vi "CommandWrite.vi"(8 "error in (no error)":errorcluster, 10 "Write Buffer":string, 11 "VISA resource name":refnum<visa-resource-name>) -> (0 "error out":errorcluster, 3 "VISA resource name out":refnum<visa-resource-name>)   [LabVIEW 2020, in "LitePoints.lvlib"]
uses:
  LitePoints.lvlib
panel:
  out "output string":string
  out "Return Count":u32
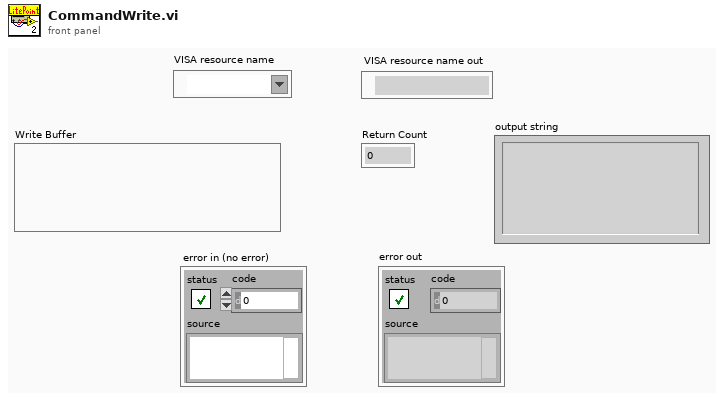
[diagram p1: front panel]
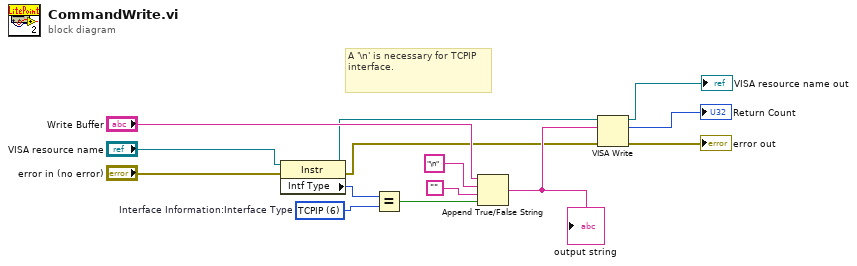
[diagram p0: block diagram]
diagram:
  w7 = u16 6 items=["GPIB"=1, "VXI"=2, "GPIB-VXI"=3, "Serial"=4, "PXI"=5, "TCPIP"=6, "USB"=7, "FireWire"=9]  # Interface Information:Interface Type
  # "A '\\n' is necessary for TCPIP interface."
  n1 = property class="Instr"(reference="VISA resource name", error in="error in (no error)") -> (reference out=w9:refnum<visa-resource-name>, error out=w2:errorcluster, "Intf Type"=w8:u16)
  n2 = Equal?(x=w8, y=w7) -> (x = y?=w6:bool)
  n3 = Append True/False String(1:w6, 2:"", 3:"\n" ("true string"), 4:"Write Buffer") -> (0:w12:string)
  "output string" <- w12
  n4 = VISA Write(VISA resource name=w9, write buffer=w12, error in (no error)=w2) -> (VISA resource name out=→"VISA resource name out":refnum<visa-resource-name>, return count=→"Return Count":u32, error out=→"error out":errorcluster)
